vi "Get Analog Edge Trigger.vi"(7 "Trigger Direction":T2, 8 "error in (no error)":errorcluster, 11 "Item Ref in":T3 format="%.0x") -> (0 "error out":errorcluster, 2 "Analog Trigger":T1, 3 "Item Ref out":T3 format="%.0x")   [LabVIEW 2012, in "Waveform Data Logger Shared.lvlib"]
uses:
  Waveform Data Logger Shared.lvlib
  <vilib>/NI Veristand/Custom Device API/Custom Device Item Ref.ctl
  Types/Trigger Direction.ctl
  Types/Analog Trigger.ctl
  Globals/Property Strings.vi
  <vilib>/NI Veristand/Custom Device API/Get Item Property (Boolean).vi
  <vilib>/NI Veristand/Custom Device API/Get Item Property (U16).vi
  <vilib>/NI Veristand/Custom Device API/Get Item Property (Double).vi
  <vilib>/NI VeriStand/Custom Device API/Custom Device API.lvlib
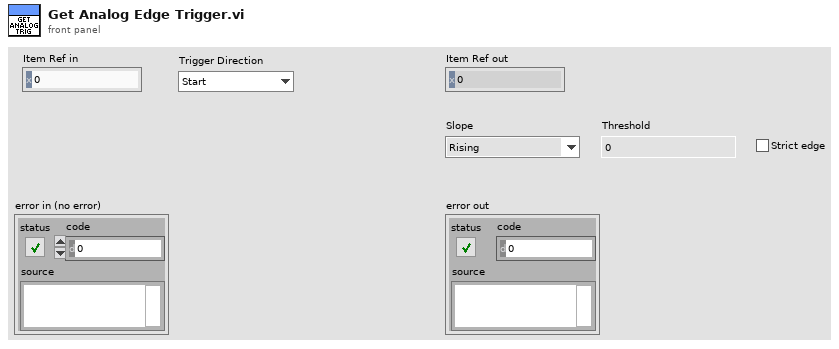
[diagram p1: front panel]
types:
  T1 = typedef "Waveform Data Logger Shared.lvlib/Analog Trigger.ctl" = cluster{"Strict edge":bool, "Slope":enum16{"Rising", "Falling"}, "Threshold":dbl}
  T2 = typedef "Waveform Data Logger Shared.lvlib/Trigger Direction.ctl" = enum16{"Start", "Stop"}
  T3 = typedef "Custom Device API.lvlib/Custom Device Item Ref.ctl" = u64
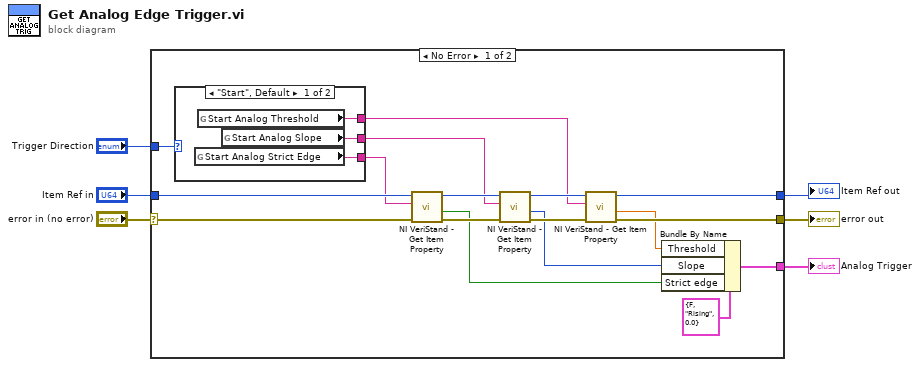
[diagram p0: block diagram]
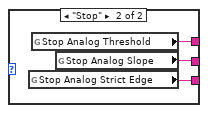
[diagram p2: hidden frame]
diagram:
  n1 = case shown="No Error" "error in (no error)" {
    selector: "error in (no error)" -> [w21 w30]
    tunnel: [w15 w31] -> w6
    tunnel: [w13 w30] -> w5
    tunnel: "Item Ref in" -> [w22 w31]
    tunnel: "Trigger Direction" -> [w23 _]
    tunnel: [w7 _] -> w1
    frame No Error {
      n2 = case shown="\"Start\", Default" w23 {
        tunnel: [w26 w28] -> w17
        tunnel: [w25 w27] -> w20
        tunnel: [w24 w29] -> w12
        frame "Start", Default {
          n3 = global read "Property Strings.vi" "Start Analog Strict Edge"() -> (w25:string)
          n4 = global read "Property Strings.vi" "Start Analog Threshold"() -> (w24:string)
          n5 = global read "Property Strings.vi" "Start Analog Slope"() -> (w26:string)
        }
        frame "Stop" {
          n6 = global read "Property Strings.vi" "Stop Analog Strict Edge"() -> (w27:string)
          n7 = global read "Property Strings.vi" "Stop Analog Threshold"() -> (w29:string)
          n8 = global read "Property Strings.vi" "Stop Analog Slope"() -> (w28:string)
        }
      }
      n9 = call-poly <vilib>:"NI VeriStand - Get Item Property.vi"("error in (no error)"=w21, "Property Name"=w20, "Item Ref in"=w22) -> ("error out"=w18:errorcluster, "Value"=w8:bool, "Item Ref out"=w19:T3)  [unwired: 1 in, 5 out]
      n10 = call-poly <vilib>:"NI VeriStand - Get Item Property.vi"("error in (no error)"=w18, "Property Name"=w17, "Item Ref in"=w19) -> ("error out"=w14:errorcluster, "Value"=w9:u16, "Item Ref out"=w16:T3)  [unwired: 1 in, 5 out]
      n11 = call-poly <vilib>:"NI VeriStand - Get Item Property.vi"("error in (no error)"=w14, "Property Name"=w12, "Item Ref in"=w16) -> ("error out"=w13:errorcluster, "Value"=w10:dbl, "Item Ref out"=w15:T3)  [unwired: 1 in, 5 out]
      n12 = Bundle By Name(cluster=T1 {"Strict edge"=FALSE, "Slope"=enum."Rising", "Threshold"=0.0} ("Analog Trigger"), "Threshold"=w10, "Slope"=w9, "Strict edge"=w8) -> (w7:T1)
    }
    frame Error {
    }
  }
  "Item Ref out" <- w6
  "error out" <- w5
  "Analog Trigger" <- w1
